vi "Initiate (Internal Buffer).vi"(8 "error in (no error)":errorcluster, 11 "VISA resource name":refnum<visa-resource-name>) -> (0 "error out":errorcluster, 3 "VISA resource name out":refnum<visa-resource-name>)   [LabVIEW 2022 SP3, in "Agilent 34401.lvlib"]
doc: "This low level VI initiates a measurement to the instrument's internal memory buffer. After you call this VI, the instrument leaves the Idle state and waits for a trigger. The readings are placed in the multimeter’s internal memory buffer. The Agilent 34401, 34410, and 34411 can hold up to <B>512, 50000, 1000000</B> readings respectively. Readings are stored until a new measurement is initiated.\n\nThis VI is intended to be used in conjunction with the <B>Fetch (Internal Buffer) VI</B>.\n\n<B>Note:</B>\n\n(1) This VI has been obsoleted from the driver and is included for compatibility with existing applications. New applications should use the <B>Initiate Measurement VI</B>.\n\n(2) This VI does not check the instrument status. Typically, you call this VI only in a sequence of calls to other low-level instrument driver VIs. The sequence performs one operation. You use the low-level VIs to optimize one or more aspects of interaction with the instrument. If you want to check the instrument status, call the <B>Error Query VI</B> at the conclusion of the sequence."
uses:
  <instrlib>/Agilent 34401/Agilent 34401.lvlib
panel:
  # "Note:\nThis VI has been obsoleted from the driver and is included for compatibility with existing applications.  New applications should use the Initiate Measurement VI."
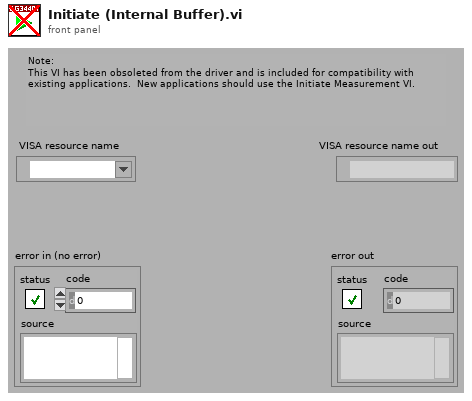
[diagram p1: front panel]
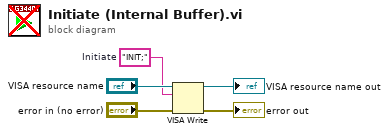
[diagram p0: block diagram]
diagram:
  w3 = "INIT;"  # Initiate
  n1 = VISA Write(VISA resource name="VISA resource name", write buffer=w3, error in (no error)="error in (no error)") -> (VISA resource name out=→"VISA resource name out":refnum<visa-resource-name>, error out=→"error out":errorcluster)  [unwired: 1 out]
